vi "Read Binary Config.vi"(4 "Class Name is Included":bool, 6 "byte order (0:big-endian, network order)":T1(ring), 8 "error in (no error)":errorcluster, 10 "Binary":string, 11 "Subset_STR in":refnum<class "Insert_STR.lvclass">) -> (0 "error out":errorcluster, 2 "Remaining":string, 3 "Subset_STR out":refnum<class "Insert_STR.lvclass">)   [LabVIEW 2021, in "Insert_STR.lvclass"]
uses:
  Insert_STR.lvclass
  Insert_STR.lvclass/Insert_STR.ctl
  Abs_Types/String/Abs_String.lvclass
  Abs_Types/Numeric/Abs_Numeric.lvclass
  Abs_Types/Value/Abs_Value.lvclass
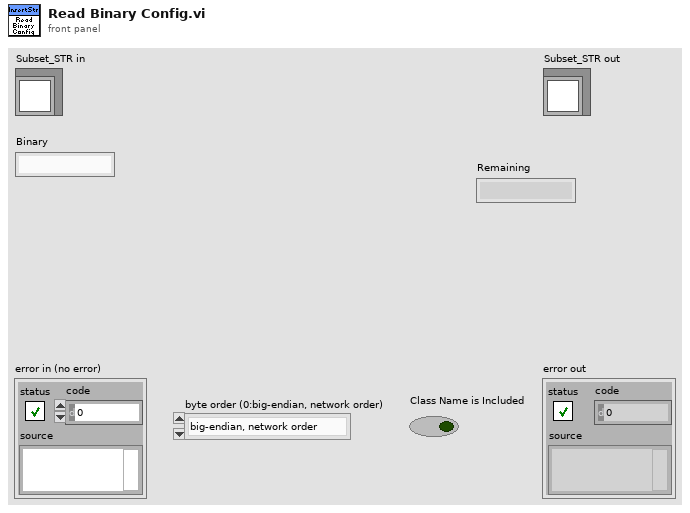
[diagram p1: front panel]
types:
  T1 = enum16{"big-endian, network order", "native, host order", "little-endian"}
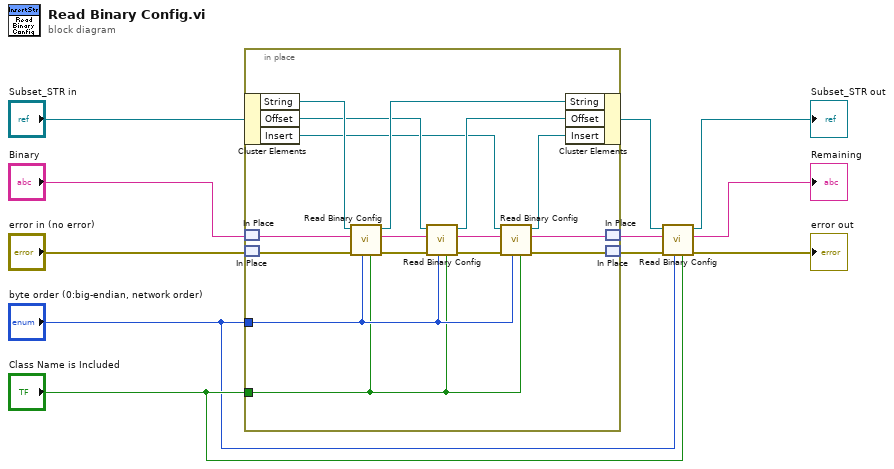
[diagram p0: block diagram]
diagram:
  n1 = in-place {
    in-place-border: "byte order (0:big-endian, network order)" -> [w13]
    in-place-border: "Class Name is Included" -> [w12]
    n2 = in-place-cluster #1("Subset_STR in") -> ("String"=w26:refnum<class "Abs_String.lvclass">, "Offset"=w21:refnum<class "Abs_Numeric.lvclass">, "Insert"=w17:refnum<class "Abs_Value.lvclass">)
    n3 = in-place-match #2("Binary") -> (w25:string)
    n4 = in-place-match #3("error in (no error)") -> (w27:errorcluster)
    n5 = call-dynamic "Read Binary Config.vi"("Class Name is Included"=w12, "byte order (0:big-endian, network order)"=w13, "error in (no error)"=w27, "Binary"=w25, "Abs_Type in"=w26) -> ("error out"=w23:errorcluster, "Remaining"=w24:string, "Abs_Type out"=w22:refnum<class "Abs_String.lvclass">)  [unwired: 4 in]
    n6 = call-dynamic "Read Binary Config.vi"("Class Name is Included"=w12, "byte order (0:big-endian, network order)"=w13, "error in (no error)"=w23, "Binary"=w24, "Abs_Type in"=w21) -> ("error out"=w19:errorcluster, "Remaining"=w18:string, "Abs_Type out"=w20:refnum<class "Abs_Numeric.lvclass">)  [unwired: 4 in]
    n7 = call-dynamic "Read Binary Config.vi"("Class Name is Included"=w12, "byte order (0:big-endian, network order)"=w13, "error in (no error)"=w19, "Binary"=w18, "Abs_Type in"=w17) -> ("error out"=w14:errorcluster, "Remaining"=w15:string, "Abs_Type out"=w16:refnum<class "Abs_Value.lvclass">)  [unwired: 4 in]
    n8 = in-place-cluster #1("String"=w22, "Offset"=w20, "Insert"=w16) -> (w2:refnum<class "Insert_STR.lvclass">)
    n9 = in-place-match #2(w15) -> (w1:string)
    n10 = in-place-match #3(w14) -> (w3:errorcluster)
  }
  n11 = call-parent "Read Binary Config.vi"("Class Name is Included"="Class Name is Included", "byte order (0:big-endian, network order)"="byte order (0:big-endian, network order)", "error in (no error)"=w3, "Binary"=w1, "Abs_Type in"=w2) -> ("error out"=→"error out":errorcluster, "Remaining"=→"Remaining":string, "Abs_Type out"=→"Subset_STR out":refnum<class "Insert_STR.lvclass">)  [unwired: 4 in]
